vi "Graph update(SubVI).vi"(6 "vy (cm/s)?":sgl, 7 "Numeric 4":dbl, 9 "Numeric in":dbl, 10 "vx (cm/s)?":sgl, 11 "milliseconds to wait":u32) -> (2 "Numeric out":dbl, 3 "Numeric 3":dbl)   [LabVIEW 2014]
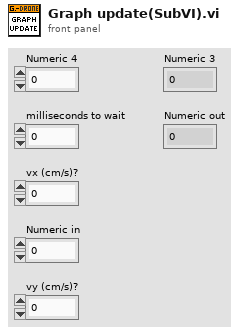
[diagram p1: front panel]
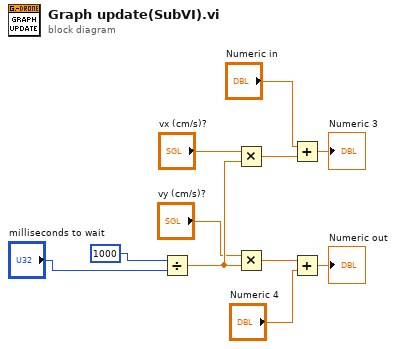
[diagram p0: block diagram]
diagram:
  n1 = Divide(x=u32 1000 ("y"), y="milliseconds to wait") -> (x/y=w11:dbl)
  n2 = Multiply(x="vx (cm/s)?", y=w11) -> (x*y=w6:dbl)
  n3 = Multiply(x="vy (cm/s)?", y=w11) -> (x*y=w8:dbl)
  n4 = Add(x="Numeric in", y=w6) -> (x+y=→"Numeric 3":dbl)
  n5 = Add(x=w8, y="Numeric 4") -> (x+y=→"Numeric out":dbl)
